vi "StahlPS_USB.ProcEvents.vi"(0 "i ref in":refnum<vi>, 5 "error in":errorcluster) -> (14 "i ref out":refnum<vi>, 19 "error out":errorcluster)   [LabVIEW 2014, in "StahlPS_USB.lvlib"]
doc: "This method is used to define the events the object will listen to. Add your own events here."
uses:
  StahlPS_USB.lvlib
  CSCore/BaseProcess/BaseProcess.event definition.ctl
  CSCore/CAEObj/CAEObj.event definition.ctl
  CSCore/BaseProcess/BaseProcess.descriptor string definition.ctl
  CSCore/BaseProcess/BaseProcess.lvlib
  CSCore/CAEObj/CAEObj.lvlib
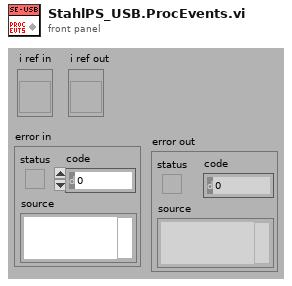
[diagram p1: front panel]
types:
  T1 = typedef "BaseProcess.lvlib/BaseProcess.event definition.ctl" = cluster{"CAEEvtDef":T2, "Data Descriptor":T3}
  T2 = typedef "CAEObj.lvlib/CAEObj.event definition.ctl" = cluster{"URL":string, "enable":bool, "ignoreResID":bool}
  T3 = typedef "BaseProcess.lvlib/BaseProcess.descriptor string definition.ctl" = string
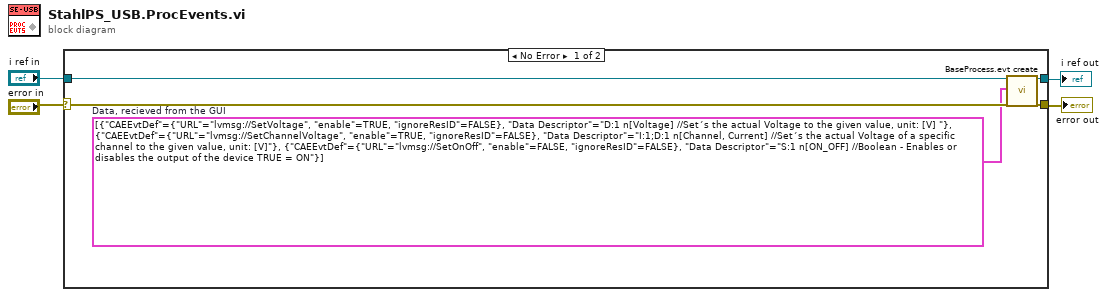
[diagram p0: block diagram]
diagram:
  n1 = case shown="No Error" "error in" {
    selector: "error in" -> [w6 w10]
    tunnel: "i ref in" -> [w7 w11]
    tunnel: [w8 w11] -> w2
    tunnel: [w9 w10] -> w1
    frame No Error {
      w5 = T1[] [{"CAEEvtDef"={"URL"="lvmsg://SetVoltage", "enable"=TRUE, "ignoreResID"=FALSE}, "Data Descriptor"="D:1 n[Voltage] //Set´s the actual Voltage to the given value, unit: [V] "}, {"CAEEvtDef"={"URL"="lvmsg://SetChannelVoltage", "enable"=TRUE, "ignoreResID"=FALSE}, "Data Descriptor"="I:1;D:1 n[Channel, Current] //Set´s the actual Voltage of a specific channel to the given value, unit: [V]"}, {"CAEEvtDef"={"URL"="lvmsg://SetOnOff", "enable"=FALSE, "ignoreResID"=FALSE}, "Data Descriptor"="S:1 n[ON_OFF] //Boolean - Enables or disables the output of the device TRUE = ON"}]  # Data, recieved from the GUI
      n2 = call "BaseProcess.evt create.vi"("i ref in"=w7, "newEvents"=w5, "error in (no error)"=w6) -> ("i ref out"=w8:refnum<vi>, "error out"=w9:errorcluster)  [unwired: 13 in, 2 out]
    }
    frame Error {
    }
  }
  "i ref out" <- w2
  "error out" <- w1
